vi "Get Worksheet.vi"(8 "error in":errorcluster, 10 "Sheet Name":string, 11 "SpreadsheetDoc in":refnum<k24>) -> (0 "error out":errorcluster, 2 "Worksheet":refnum<k24>, 3 "SpreadsheetDoc out":refnum<k24>, 5 "SheetName":string)   [LabVIEW 2019, in "Open Xml.lvlib"]
uses:
  Open Xml.lvlib
  D:/git/Open-Xml-LabVIEW/Source/DocumentFormat.OpenXml.dll
  DocumentFormat.OpenXml.dll
  D:/git/Open-Xml-LabVIEW/Source/DocumentFormat.OpenXml.Framework.dll
  DocumentFormat.OpenXml.Framework.dll
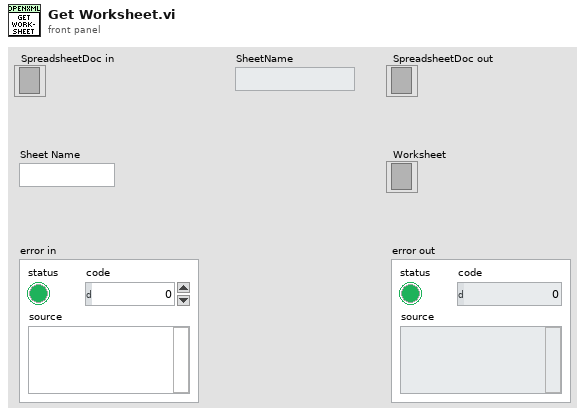
[diagram p1: front panel]
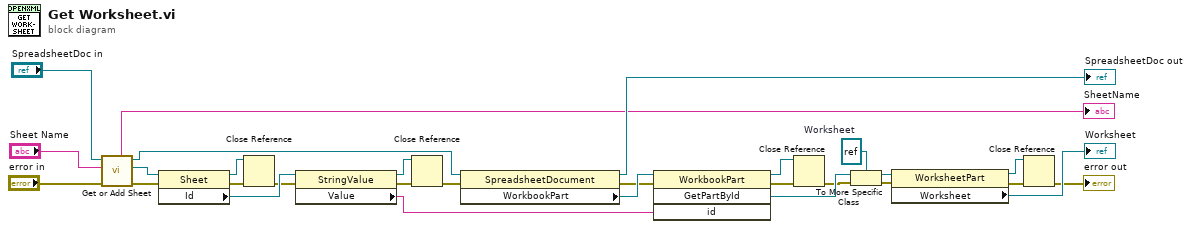
[diagram p0: block diagram]
diagram:
  w11 = refnum<k24> refnum  # Worksheet
  n1 = call "Get or Add Sheet.vi"("error in"="error in", "Sheet Name"="Sheet Name", "SpreadsheetDoc in"="SpreadsheetDoc in") -> ("error out"=w20:errorcluster, "Sheet"=w19:refnum<k24>, "SpreadsheetDoc out"=w26:refnum<k24>, "SheetName"=→"SheetName":string)  [unwired: 4 in, 1 out]
  n2 = property class="Sheet"(reference=w19, error in=w20) -> (reference out=w14:refnum<k24>, error out=w21:errorcluster, "Id"=w22:refnum<k24>)
  n3 = Close Reference(reference=w14, error in (no error)=w21) -> (error out=w15:errorcluster)
  n4 = property class="StringValue"(reference=w22, error in=w15) -> (reference out=w9:refnum<k24>, error out=w17:errorcluster, "Value"=w18:string)
  n5 = Close Reference(reference=w9, error in (no error)=w17) -> (error out=w10:errorcluster)
  n6 = property class="SpreadsheetDocument"(reference=w26, error in=w10) -> (reference out=→"SpreadsheetDoc out":refnum<k24>, error out=w24:errorcluster, "WorkbookPart"=w25:refnum<k24>)
  n7 = invoke class="WorkbookPart" method="GetPartById"(reference=w25, error in=w24, "id"=w18) -> (reference out=w7:refnum<k24>, error out=w23:errorcluster, "GetPartById"=w12:refnum<k24>)  [unwired: 1 in, 1 out]
  n8 = Close Reference(reference=w7, error in (no error)=w23) -> (error out=w8:errorcluster)
  n9 = To More Specific Class(target class=w11, reference=w12, error in=w8) -> (specific class reference=w5:refnum<k24>, error out=w13:errorcluster)
  n10 = property class="WorksheetPart"(reference=w5, error in=w13) -> (reference out=w1:refnum<k24>, error out=w2:errorcluster, "Worksheet"=→"Worksheet":refnum<k24>)
  n11 = Close Reference(reference=w1, error in (no error)=w2) -> (error out=→"error out":errorcluster)
